vi "rsscope_quotedInt_WriteCallback.vi"(5 "Attribute":T1={"Identifier"="", "Descriptive Name"="", "Data Type"=enum."Integer 32", "Command"="", "Access"=enum."Read/Write", "Range Table"="", "Read Callback"="", "Write Callback"="", "Supported Models"="", "Instrument Options"="", "Index"=0, "OPC Wait"=FALSE, "No Status Check"=FALSE, "Cache Only"=FALSE}, 7 "Repeated Capability":string="Win1", 8 "error in (no error)":errorcluster, 10 "Attribute Value I32":i32, 11 "VISA resource name":refnum<visa-resource-name>) -> (0 "error out":errorcluster, 3 "VISA resource name out":refnum<visa-resource-name>)   [LabVIEW 2014]
uses:
  rsidr_core.llb/rsscope_rsidr_core.lvlib
  rsidr_core.llb/type_Attribute_Data_Type.ctl
  rsidr_core.llb/type_Attribute.ctl
  rsidr_core.llb/type_ReadWriteAccess.ctl
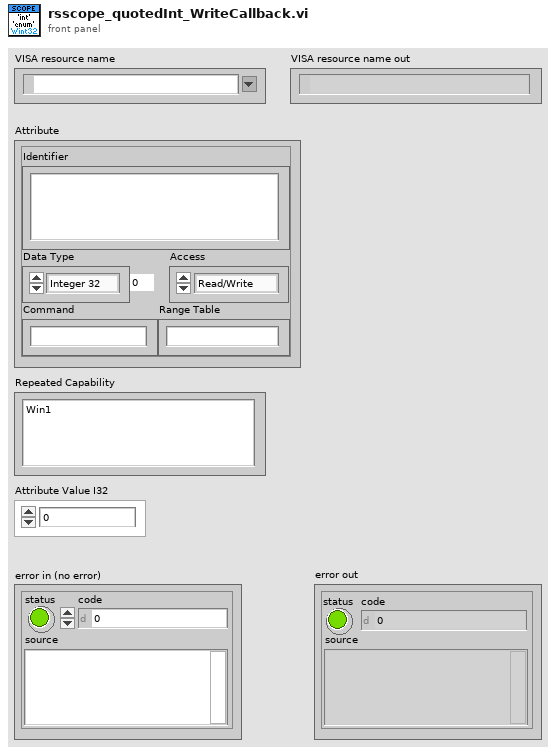
[diagram p1: front panel]
types:
  T1 = typedef "rsscope_rsidr_core.lvlib/type_Attribute.ctl" = cluster{"Identifier":string, "Descriptive Name":string, "Data Type":T2, "Command":string, "Access":T3, "Range Table":string, "Read Callback":string, "Write Callback":string, "Supported Models":string, "Instrument Options":string, "Index":i32, "OPC Wait":bool, "No Status Check":bool, "Cache Only":bool}
  T2 = typedef "rsscope_rsidr_core.lvlib/type_Attribute_Data_Type.ctl" = enum16{"Integer 32", "Double", "String", "Boolean", "None", "Integer 64", "RawString"}
  T3 = typedef "rsscope_rsidr_core.lvlib/type_ReadWriteAccess.ctl" = enum16{"Read Only", "Write Only", "Read/Write"}
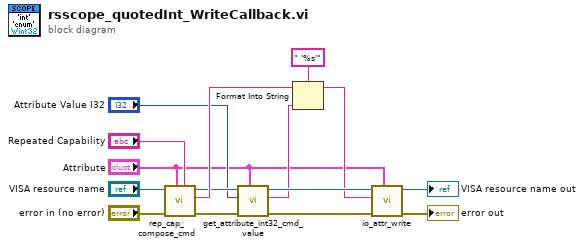
[diagram p0: block diagram]
diagram:
  n1 = call "rep_cap_compose_cmd.vi"("Repeated Capability"="Repeated Capability", "Attribute"="Attribute", "error in"="error in (no error)", "VISA resource name"="VISA resource name") -> ("error out"=w12:errorcluster, "Command out"=w15:string, "VISA resource name out"=w13:refnum<visa-resource-name>)  [unwired: 5 in]
  n2 = call "get_attribute_int32_cmd_value.vi"("Attribute"="Attribute", "error in"=w12, "Input Int32 value"="Attribute Value I32", "VISA resource name"=w13) -> ("error out"=w9:errorcluster, "Cmd Value out"=w2:string, "VISA resource name out"=w8:refnum<visa-resource-name>)  [unwired: 5 in]
  n3 = Format Into String(format string=" '%s'", initial string=w15, w2) -> (resulting string=w7:string)  [unwired: 1 in, 1 out]
  n4 = call "io_attr_write.vi"("Attribute"="Attribute", "error in"=w9, "write buffer"=w7, "VISA resource name"=w8) -> ("error out"=→"error out":errorcluster, "VISA resource name out"=→"VISA resource name out":refnum<visa-resource-name>)  [unwired: 6 in]
